vi "Teleop.vi"(10 "Match Info":T1={"Autonomous Elapsed Seconds"=0.0, "TeleOp Elapsed Seconds"=0.0, "Disabled Elapsed Seconds"=0.0, "Visited Autonomous"=FALSE, "Visited TeleOp"=FALSE, "Visited Disabled"=FALSE, "Autonomous Settings"={"Autonomous Style"=enum."Independent", "VI Refnum"=refnum}}, 11 "Call Context":T2) -> ()   [LabVIEW 2016]
doc: "This VI is called for each TeleOp packet received from the DS where the robot is not disabled. It is often used to read from the joysticks and update I/O or to update setpoints for timed control loops. It should complete and return within 20 milliseconds or it may miss DS packets."
uses:
  <vilib>/Rock Robotics/WPI/DriverStation/WPI_DriverStationDerivedRobotMode.ctl
  <vilib>/Rock Robotics/WPI/DriverStation/WPI_DriverStationMatch Info.ctl
  <vilib>/Rock Robotics/WPI/Relay/WPI_RelayValue.ctl
  <vilib>/Rock Robotics/WPI/Utilities/WPI_GetSetVariantRefNum.vi
  <vilib>/Rock Robotics/Network Tables/NT Write Boolean.vi
  <vilib>/Rock Robotics/Network Tables/NT Read Boolean.vi
  <vilib>/Rock Robotics/Network Tables/NT Read Number.vi
  AutoaimVar.vi
panel:
  out "r button pressed?":bool
  out "Sample Slider 0":dbl(slide) scale=0.0..5.0
  out "Sample Boolean 1":bool
  out "Sample Boolean 0":bool
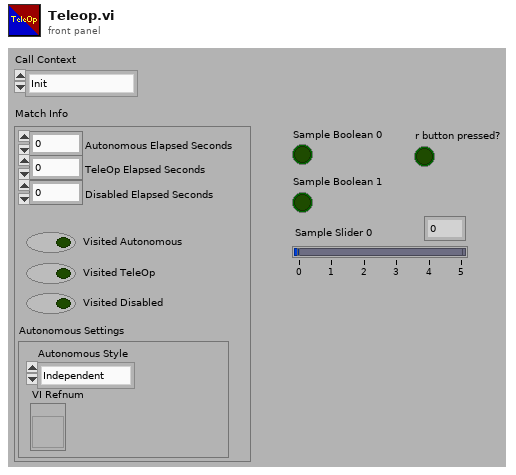
[diagram p1: front panel]
types:
  T1 = typedef "WPI_DriverStationMatch Info.ctl" = cluster{"Autonomous Elapsed Seconds":dbl, "TeleOp Elapsed Seconds":dbl, "Disabled Elapsed Seconds":dbl, "Visited Autonomous":bool, "Visited TeleOp":bool, "Visited Disabled":bool, "Autonomous Settings":cluster{"Autonomous Style":enum16{"Iterative", "Independent"}, "VI Refnum":refnum<vi>}}
  T2 = typedef "WPI_DriverStationDerivedRobotMode.ctl" = enum16{"Init", "Execute", "Stop"}
  T3 = typedef "WPI_JoystickDevRef.ctl" = cluster{"Device":T4}
  T4 = typedef "WPI_JoystickDeviceEnum.ctl" = enum16{"USB 0", "USB 1", "USB 2", "USB 3", "USB 4", "USB 5"}
  T5 = typedef "WPI_RelayValue.ctl" = enum16{"Off", "On", "Forward", "Reverse"}
  T6 = typedef "WPI_RelayDevRef.ctl" = cluster{"DevStatus":errorcluster, "Relay Channel":T7, "Relay Direction":T8}
  T7 = typedef "FPGA_DIORelayChannel.ctl" = enum8{"Relay 0", "Relay 1", "Relay 2", "Relay 3", "Invalid"}
  T8 = typedef "WPI_RelayDirection.ctl" = enum16{"Both directions", "Forward only", "Reverse only"}
  T9 = typedef "WPI_MotorControlDeviceRef.ctl" = cluster{"DeviceStatus":errorcluster, "Type":T10, "PWM":cluster{"PWM Channel":T11, "DeadBand":T12}, "CAN":cluster{"Device Number":u8, "SetOutput VI Ref":variant, "GetOutput VI Ref":variant, "Enable VI Ref":variant, "Disable VI Ref":variant, "Data":variant}, "Invert":bool}
  T10 = typedef "WPI_MotorControlType.ctl" = enum16{"PWM", "CAN"}
  T11 = typedef "FPGA_DIOPWMChannel.ctl" = enum8{"PWM 0", "PWM 1", "PWM 2", "PWM 3", "PWM 4", "PWM 5", "PWM 6", "PWM 7", "PWM 8", "PWM 9", "PWM MXP 0", "PWM MXP 1", "PWM MXP 2", "PWM MXP 3", "PWM MXP 4", "PWM MXP 5", "PWM MXP 6", "PWM MXP 7", "PWM MXP 8", "PWM MXP 9", "Invalid"}
  T12 = typedef "WPI_PWMDeadband.ctl" = cluster{"Name":string, "maxPositivePwm":i32, "minPositivePwm":i32, "centerPwm":i32, "maxNegativePwm":i32, "minNegativePwm":i32, "angularRange":u16}
  T13 = typedef "WPI_RobotDriveDevRef.ctl" = cluster{"DevStatus":errorcluster, "Motors[]":T9[], "Square Inputs":bool, "Max Output":dbl}
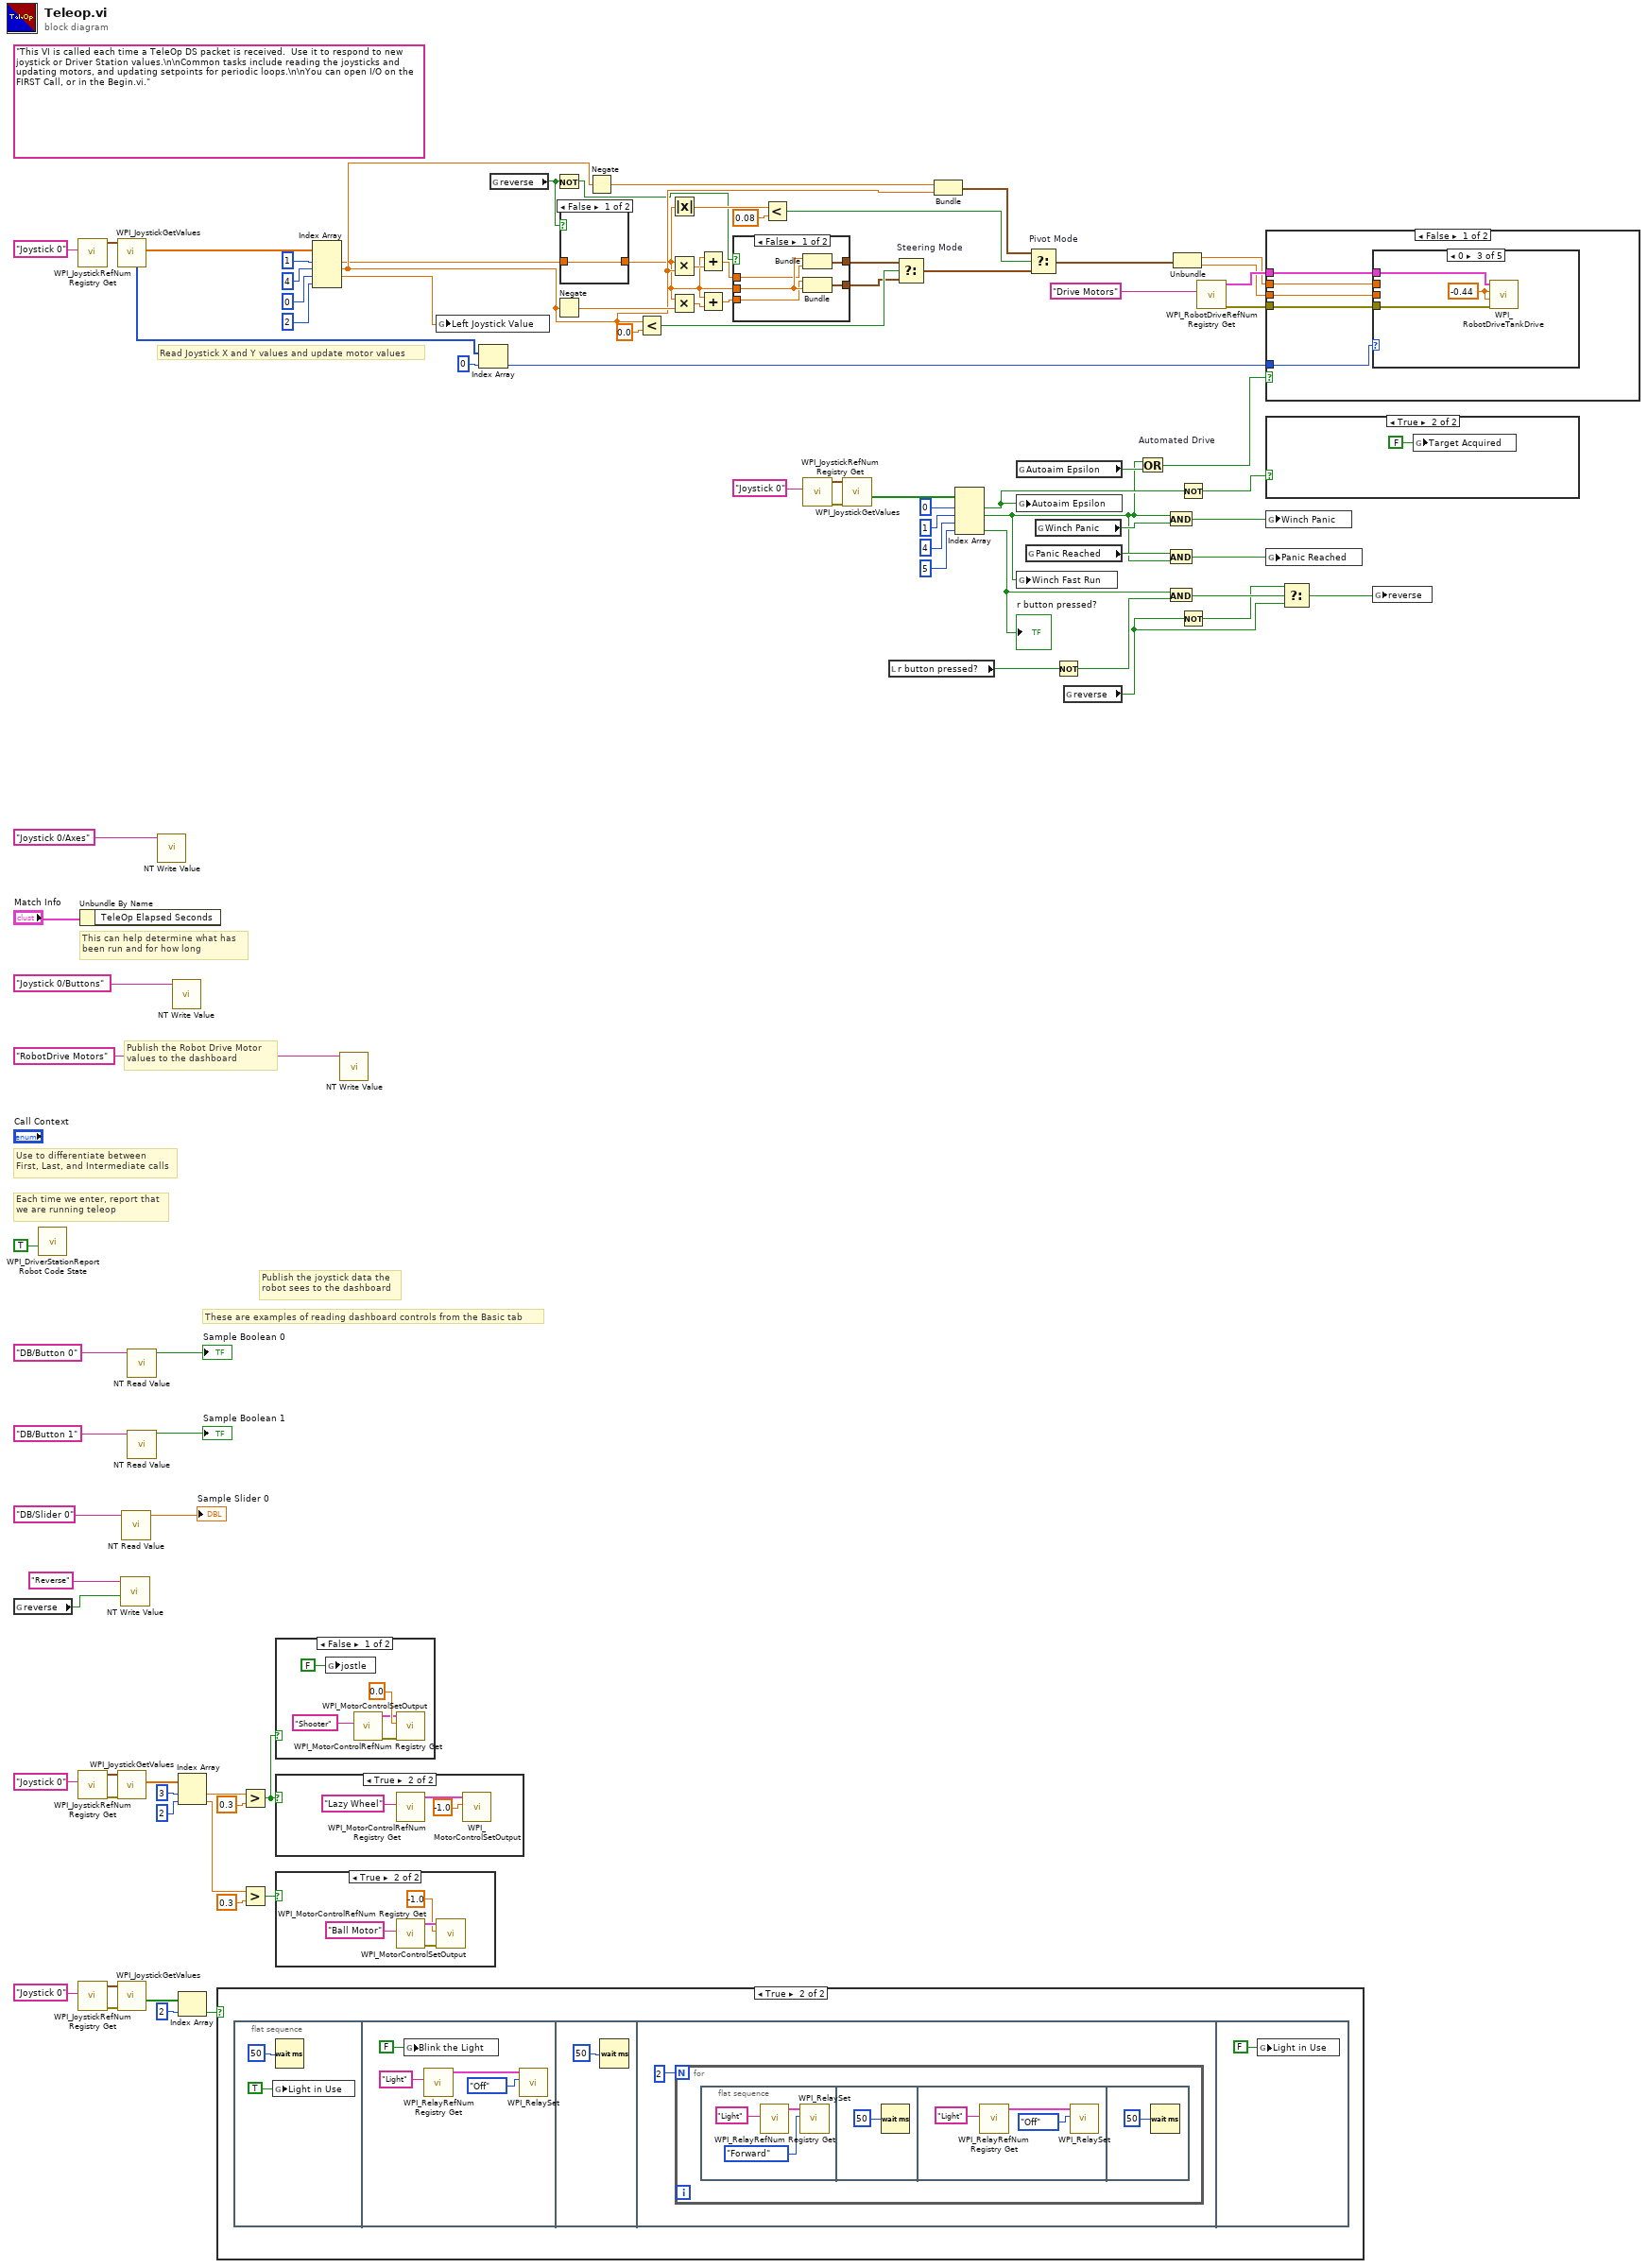
[diagram p0: block diagram]
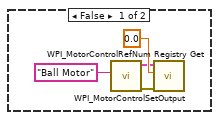
[diagram p3: hidden frame]
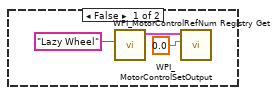
[diagram p4: hidden frame]
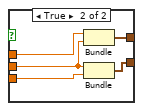
[diagram p5: hidden frame]
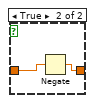
[diagram p6: hidden frame]
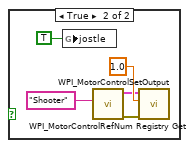
[diagram p7: hidden frame]
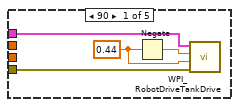
[diagram p9: hidden frame]
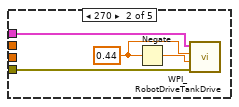
[diagram p10: hidden frame]
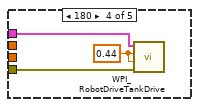
[diagram p11: hidden frame]
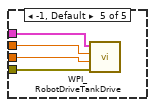
[diagram p12: hidden frame]
diagram:
  (unwired) "This VI is called each time a TeleOp DS packet is received.  Use it to respond to new joystick or Driver Station values.\n\nCommon tasks include reading the joysticks and updating motors, and updating setpoints for periodic loops.\n\nYou can open I/O on the FIRST Call, or in the Begin.vi."
  # "These are examples of reading dashboard controls from the Basic tab"
  # "Publish the Robot Drive Motor\nvalues to the dashboard"
  # "Publish the joystick data the\nrobot sees to the dashboard"
  # "Each time we enter, report that\nwe are running teleop"
  # "Use to differentiate between\nFirst, Last, and Intermediate calls"
  # "This can help determine what has\nbeen run and for how long"
  # "Read Joystick X and Y values and update motor values"
  n1 = global read "AutoaimVar.vi" "reverse"() -> (w26:bool)
  n2 = call <vilib>:"WPI_DriverStationReport Robot Code State.vi"("TeleOp"=TRUE ("Autonomous")) -> ()  [unwired: 10 in, 1 out]
  n3 = call <vilib>:"WPI_JoystickRefNum Registry Get.vi"("refnum name"="Joystick 0") -> ("JoystickDevRef"=w74:T3)  [unwired: 1 in, 9 out]
  n4 = call <vilib>:"WPI_JoystickRefNum Registry Get.vi"("refnum name"="Joystick 0") -> ("error out"=w22:errorcluster, "JoystickDevRef"=w21:T3)  [unwired: 9 in]
  n5 = call <vilib>:"WPI_JoystickRefNum Registry Get.vi"("refnum name"="Joystick 0") -> ("error out"=w5:errorcluster, "JoystickDevRef"=w7:T3)  [unwired: 9 in]
  n6 = Unbundle By Name("Match Info") -> ()  [unwired: 1 out]
  n7 = call <vilib>:"WPI_JoystickGetValues.vi"("JoystickDevRef"=w74) -> ("Axes"=w71:dbl[], "POVs"=w10:i16[])  [unwired: 6 in, 3 out]
  n8 = call <vilib>:"WPI_JoystickGetValues.vi"("error in (no error)"=w22, "JoystickDevRef"=w21) -> ("Axes"=w18:dbl[])  [unwired: 5 in, 4 out]
  n9 = call <vilib>:"WPI_JoystickGetValues.vi"("error in (no error)"=w5, "JoystickDevRef"=w7) -> ("Buttons"=w4:bool[])  [unwired: 5 in, 4 out]
  n10 = call-poly <vilib>:"NT Write Value.vi"("Boolean"=w26, "Name"="Reverse") -> ()  [unwired: 9 in, 1 out]
  n11 = call-poly <vilib>:"NT Read Value.vi"("Name"="DB/Slider 0" ("refnum name")) -> ("Numeric"=→"Sample Slider 0":dbl)  [unwired: 9 in, 1 out]
  n12 = call-poly <vilib>:"NT Read Value.vi"("Name"="DB/Button 0" ("refnum name")) -> ("Boolean"=→"Sample Boolean 0":bool)  [unwired: 9 in, 1 out]
  n13 = call-poly <vilib>:"NT Read Value.vi"("Name"="DB/Button 1" ("refnum name")) -> ("Boolean"=→"Sample Boolean 1":bool)  [unwired: 9 in, 1 out]
  n14 = call-poly <vilib>:"NT Write Value.vi"("Name"="Joystick 0/Axes") -> ()  [unwired: 10 in, 1 out]
  n15 = call-poly <vilib>:"NT Write Value.vi"("Name"="Joystick 0/Buttons") -> ()  [unwired: 10 in, 1 out]
  n16 = Index Array(array=w18, index #1=3 ("index"), index #2=2 ("index")) -> (element #1=w17:dbl, element #2=w11:dbl)
  n17 = Index Array(array=w4, index=2) -> (element=w2:bool)
  n18 = case shown="True" w2 {
    frame False {
    }
    frame True {
      n19 = flat-sequence {
        frame #0 {
          n20 = global write "AutoaimVar.vi" "Light in Use"(TRUE ("Light in Use")) -> ()
          n21 = Wait (ms)(milliseconds to wait=u32 50) -> ()  [unwired: 1 out]
        }
        frame #1 {
          n22 = global write "AutoaimVar.vi" "Blink the Light"(FALSE ("Blink the Light")) -> ()
          n23 = call <vilib>:"WPI_RelayRefNum Registry Get.vi"("refnum name"="Light") -> ("RelayDevRef"=w95:T6)  [unwired: 9 in, 1 out]
          n24 = call <vilib>:"WPI_RelaySet.vi"("RelayValue"=WPI_RelayValue."Off", "RelayDevRef"=w95) -> ()  [unwired: 8 in, 2 out]
        }
        frame #2 {
          n25 = Wait (ms)(milliseconds to wait=u32 50) -> ()  [unwired: 1 out]
        }
        frame #3 {
          n26 = for {
            N: 2 -> [_]
            n27 = flat-sequence {
              frame #0 {
                n28 = call <vilib>:"WPI_RelayRefNum Registry Get.vi"("refnum name"="Light") -> ("RelayDevRef"=w103:T6)  [unwired: 9 in, 1 out]
                n29 = call <vilib>:"WPI_RelaySet.vi"("RelayValue"=WPI_RelayValue."Forward", "RelayDevRef"=w103) -> ()  [unwired: 8 in, 2 out]
              }
              frame #1 {
                n30 = Wait (ms)(milliseconds to wait=u32 50) -> ()  [unwired: 1 out]
              }
              frame #2 {
                n31 = call <vilib>:"WPI_RelayRefNum Registry Get.vi"("refnum name"="Light") -> ("RelayDevRef"=w107:T6)  [unwired: 9 in, 1 out]
                n32 = call <vilib>:"WPI_RelaySet.vi"("RelayValue"=WPI_RelayValue."Off", "RelayDevRef"=w107) -> ()  [unwired: 8 in, 2 out]
              }
              frame #3 {
                n33 = Wait (ms)(milliseconds to wait=u32 50) -> ()  [unwired: 1 out]
              }
            }
          }
        }
        frame #4 {
          n34 = global write "AutoaimVar.vi" "Light in Use"(FALSE ("Light in Use")) -> ()
        }
      }
    }
  }
  n35 = Greater?(x=w17, y=0.3) -> (0:w15:bool)
  n36 = Greater?(x=w11, y=0.3) -> (0:w12:bool)
  n37 = case shown="False" w15 {
    frame False {
      n38 = global write "AutoaimVar.vi" "jostle"(FALSE ("jostle")) -> ()
      n39 = call <vilib>:"WPI_MotorControlRefNum Registry Get.vi"("refnum name"="Shooter") -> ("error out"=w111:errorcluster, "MotorControlDevRef"=w112:T9)  [unwired: 9 in]
      n40 = call <vilib>:"WPI_MotorControlSetOutput.vi"("error in (no error)"=w111, "Output"=0.0, "MotorControlDevRef"=w112) -> ()  [unwired: 6 in, 3 out]
    }
    frame True {
      n41 = global write "AutoaimVar.vi" "jostle"(TRUE ("jostle")) -> ()
      n42 = call <vilib>:"WPI_MotorControlRefNum Registry Get.vi"("refnum name"="Shooter") -> ("error out"=w116:errorcluster, "MotorControlDevRef"=w117:T9)  [unwired: 9 in]
      n43 = call <vilib>:"WPI_MotorControlSetOutput.vi"("error in (no error)"=w116, "Output"=1.0, "MotorControlDevRef"=w117) -> ()  [unwired: 6 in, 3 out]
    }
  }
  n44 = case shown="True" w15 {
    frame False {
      n45 = call <vilib>:"WPI_MotorControlRefNum Registry Get.vi"("refnum name"="Lazy Wheel") -> ("MotorControlDevRef"=w121:T9)  [unwired: 9 in, 1 out]
      n46 = call <vilib>:"WPI_MotorControlSetOutput.vi"("Output"=0.0, "MotorControlDevRef"=w121) -> ()  [unwired: 7 in, 3 out]
    }
    frame True {
      n47 = call <vilib>:"WPI_MotorControlRefNum Registry Get.vi"("refnum name"="Lazy Wheel") -> ("MotorControlDevRef"=w124:T9)  [unwired: 9 in, 1 out]
      n48 = call <vilib>:"WPI_MotorControlSetOutput.vi"("Output"=-1.0, "MotorControlDevRef"=w124) -> ()  [unwired: 7 in, 3 out]
    }
  }
  n49 = case shown="True" w12 {
    frame False {
      n50 = call <vilib>:"WPI_MotorControlRefNum Registry Get.vi"("refnum name"="Ball Motor") -> ("error out"=w129:errorcluster, "MotorControlDevRef"=w126:T9)  [unwired: 9 in]
      n51 = call <vilib>:"WPI_MotorControlSetOutput.vi"("error in (no error)"=w129, "Output"=0.0, "MotorControlDevRef"=w126) -> ()  [unwired: 6 in, 3 out]
    }
    frame True {
      n52 = call <vilib>:"WPI_MotorControlRefNum Registry Get.vi"("refnum name"="Ball Motor") -> ("error out"=w131:errorcluster, "MotorControlDevRef"=w132:T9)  [unwired: 9 in]
      n53 = call <vilib>:"WPI_MotorControlSetOutput.vi"("error in (no error)"=w131, "Output"=-1.0, "MotorControlDevRef"=w132) -> ()  [unwired: 6 in, 3 out]
    }
  }
  n54 = Index Array(array=w71, index #1=1 ("index"), index #2=4 ("index"), index #3=0 ("index"), index #4=2 ("index")) -> (element #1=w29:dbl, element #2=w54:dbl, element #3=w41:dbl)  [unwired: 1 out]
  n55 = call-poly <vilib>:"NT Write Value.vi"("Name"="RobotDrive Motors") -> ()  [unwired: 10 in, 1 out]
  n56 = global write "AutoaimVar.vi" "Left Joystick Value"(w41) -> ()
  n57 = Index Array(array=w10, index=0) -> (element=w8:i16)
  n58 = global read "AutoaimVar.vi" "reverse"() -> (w25:bool)
  n59 = Not(x=w25) -> (.not. x?=w24:bool)
  n60 = Negate(x=w54) -> (-x=w69:dbl)
  n61 = case shown="False" w25 {
    tunnel: w29 -> [w134 w136]
    tunnel: [w134 w135] -> w28
    frame False {
    }
    frame True {
      n62 = Negate(x=w136) -> (-x=w135:dbl)
    }
  }
  n63 = Negate(x=w54) -> (-x=w55:dbl)
  n64 = Less?(x=w54, y=0.0) -> (x < y?=w64:bool)
  n65 = Absolute Value(x=w28) -> (abs(x)=w61:dbl)
  n66 = Multiply(x=w28, y=w54) -> (x*y=w70:dbl)
  n67 = Multiply(x=w28, y=w69) -> (x*y=w68:dbl)
  n68 = Add(x=w28, y=w70) -> (x+y=w66:dbl)
  n69 = Add(x=w28, y=w68) -> (x+y=w65:dbl)
  n70 = case shown="False" w24 {
    tunnel: w66 -> [w140 w146]
    tunnel: w65 -> [w139 w145]
    tunnel: [w138 w144] -> w63
    tunnel: [w137 w143] -> w62
    tunnel: w28 -> [w141 w142]
    frame False {
      n71 = Bundle("upper limit"=w141, w140) -> (w138:cluster{"upper limit":dbl, dbl})  [unwired: 1 in]
      n72 = Bundle(w139, "upper limit"=w141) -> (w137:cluster{dbl, "upper limit":dbl})  [unwired: 1 in]
    }
    frame True {
      n73 = Bundle(w146, "upper limit"=w142) -> (w144:cluster{dbl, "upper limit":dbl})  [unwired: 1 in]
      n74 = Bundle("upper limit"=w142, w145) -> (w143:cluster{"upper limit":dbl, dbl})  [unwired: 1 in]
    }
  }
  n75 = Less?(x=w61, y=0.08) -> (x < y?=w59:bool)
  n76 = call <vilib>:"WPI_JoystickRefNum Registry Get.vi"("refnum name"="Joystick 0") -> ("error out"=w78:errorcluster, "JoystickDevRef"=w80:T3)  [unwired: 9 in]
  n77 = call <vilib>:"WPI_JoystickGetValues.vi"("error in (no error)"=w78, "JoystickDevRef"=w80) -> ("Buttons"=w76:bool[])  [unwired: 5 in, 4 out]
  n78 = local read "r button pressed?"() -> (w32:bool)
  n79 = Select "Steering Mode"(t=w63, s=w64, f=w62) -> (s? t:f=w58:cluster{"upper limit":dbl, "upper limit":dbl})
  n80 = Bundle(w55, "upper limit"=w54) -> (w57:cluster{dbl, "upper limit":dbl})  [unwired: 1 in]
  n81 = Index Array(array=w76, index #1=0 ("index"), index #2=1 ("index"), index #3=4 ("index"), index #4=5 ("index")) -> (element #1=w48:bool, element #2=w38:bool, element #4=w35:bool)  [unwired: 1 out]
  "r button pressed?" <- w35
  n82 = global read "AutoaimVar.vi" "Autoaim Epsilon"() -> (w40:bool)
  n83 = global write "AutoaimVar.vi" "Autoaim Epsilon"(w48) -> ()
  n84 = global write "AutoaimVar.vi" "Winch Fast Run"(w38) -> ()
  n85 = global read "AutoaimVar.vi" "Panic Reached"() -> (w44:bool)
  n86 = Select "Pivot Mode"(t=w57, s=w59, f=w58) -> (s? t:f=w56:cluster{"upper limit":dbl, "upper limit":dbl})
  n87 = global read "AutoaimVar.vi" "Winch Panic"() -> (w46:bool)
  n88 = Not(x=w32) -> (.not. x?=w36:bool)
  n89 = global read "AutoaimVar.vi" "reverse"() -> (w30:bool)
  n90 = Or "Automated Drive"(x=w38, y=w40) -> (x .or. y?=w39:bool)
  n91 = And(x=w38, y=w46) -> (x .and. y?=w45:bool)
  n92 = And(x=w44, y=w38) -> (x .and. y?=w43:bool)
  n93 = And(x=w35, y=w36) -> (x .and. y?=w34:bool)
  n94 = Unbundle(w56) -> ("upper limit"=w49:dbl, "upper limit"=w51:dbl)
  n95 = Not(x=w48) -> (.not. x?=w47:bool)
  n96 = Not(x=w30) -> (.not. x?=w31:bool)
  n97 = call <vilib>:"WPI_RobotDriveRefNum Registry Get.vi"("refnum name"="Drive Motors") -> ("error out"=w52:errorcluster, "RobotDriveDevRef"=w53:T13)  [unwired: 1 in, 8 out]
  n98 = case shown="False" w39 {
    tunnel: w53 -> [w151 _]
    tunnel: w52 -> [w150 _]
    tunnel: w51 -> [w149 _]
    tunnel: w49 -> [w148 _]
    tunnel: w8 -> [w147 _]
    frame False {
      n99 = case shown="0" w147 {
        tunnel: w151 -> [w155 w158 w161 w164 w169]
        tunnel: w150 -> [w154 w159 w162 w163 w168]
        tunnel: w149 -> [_ _ _ _ w166]
        tunnel: w148 -> [_ _ _ _ w167]
        frame 90 {
          w153 = 0.44 ("Right axis value")
          n100 = Negate(x=w153) -> (-x=w152:dbl)
          n101 = call <vilib>:"WPI_RobotDriveTankDrive.vi"("error in (no error)"=w154, "Right axis value"=w153, "Left axis value"=w152, "RobotDriveDevRef"=w155) -> ()  [unwired: 5 in, 3 out]
        }
        frame 270 {
          w156 = 0.44 ("Right axis value")
          n102 = Negate(x=w156) -> (-x=w157:dbl)
          n103 = call <vilib>:"WPI_RobotDriveTankDrive.vi"("error in (no error)"=w159, "Right axis value"=w157, "Left axis value"=w156, "RobotDriveDevRef"=w158) -> ()  [unwired: 5 in, 3 out]
        }
        frame 0 {
          w160 = -0.44 ("Right axis value")
          n104 = call <vilib>:"WPI_RobotDriveTankDrive.vi"("error in (no error)"=w162, "Right axis value"=w160, "Left axis value"=w160, "RobotDriveDevRef"=w161) -> ()  [unwired: 5 in, 3 out]
        }
        frame 180 {
          w165 = 0.44 ("Right axis value")
          n105 = call <vilib>:"WPI_RobotDriveTankDrive.vi"("error in (no error)"=w163, "Right axis value"=w165, "Left axis value"=w165, "RobotDriveDevRef"=w164) -> ()  [unwired: 5 in, 3 out]
        }
        frame -1, Default {
          n106 = call <vilib>:"WPI_RobotDriveTankDrive.vi"("error in (no error)"=w168, "Right axis value"=w166, "Left axis value"=w167, "RobotDriveDevRef"=w169) -> ()  [unwired: 5 in, 3 out]
        }
      }
    }
    frame True {
    }
  }
  n107 = case shown="True" w47 {
    frame False {
    }
    frame True {
      n108 = global write "AutoaimVar.vi" "Target Acquired"(FALSE ("Target Acquired")) -> ()
    }
  }
  n109 = global write "AutoaimVar.vi" "Winch Panic"(w45) -> ()
  n110 = global write "AutoaimVar.vi" "Panic Reached"(w43) -> ()
  n111 = Select(t=w31, s=w34, f=w30) -> (s? t:f=w33:bool)
  n112 = global write "AutoaimVar.vi" "reverse"(w33) -> ()
